vi "Timeout AutoKAL.vi"(6 "Aktionen":T1) -> (0 "Timeout":bool, 2 "Verstrichene Zeit":dbl)   [LabVIEW 2020, in "Auto Kalibrieren.lvlib"]
uses:
  Auto Kalibrieren.lvlib
  Aktionen Timeout.ctl
  Aktionen FGV Zustand Kalibrierung.ctl
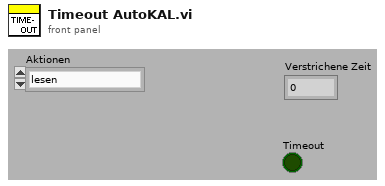
[diagram p1: front panel]
types:
  T1 = typedef "Auto Kalibrieren.lvlib/Aktionen Timeout.ctl" = enum16{"lesen", "init", "prüfen"}
  T2 = typedef "Auto Kalibrieren.lvlib/Aktionen FGV Zustand Kalibrierung.ctl" = enum16{"lesen", "LÖSCHEN", "Hintergrund fertig", "Nullpunkt NDIR CO lo", "Endpunkt NDIR CO lo", "Nullpunkt NDIR CO hi", "Endpunkt NDIR CO hi", "Nullpunkt NDIR CO2 lo", "Endpunkt NDIR CO2 lo", "Nullpunkt FID CH4", "Endpunkt FID CH4", "Nullpunkt FID THC", "Endpunkt FID THC", "Nullpunkt PMA", "Endpunkt PMA", "Fehler FT-IR", "Fehler NDIR lo", "Fehler FID CH4", "Fehler FID THC", "Fehler PMA", "TIMEOUT"}
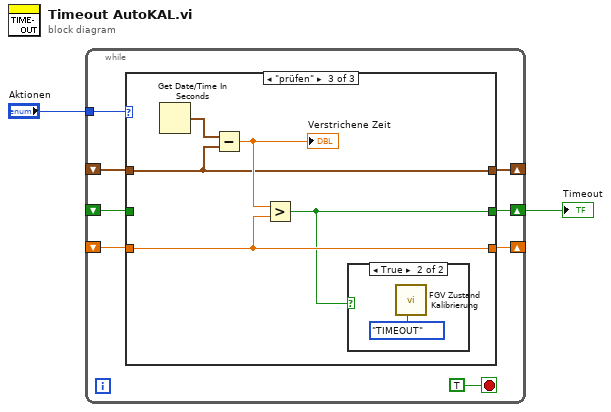
[diagram p0: block diagram]
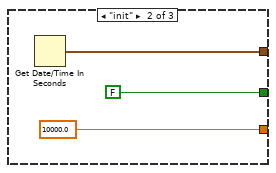
[diagram p3: hidden frame]
diagram:
  n1 = while {
    tunnel: "Aktionen" -> [w9]
    shift-right: [w8] -> _
    shift-left: _ -> [w7]
    shift-right: [w5] -> _
    shift-left: _ -> [w6]
    shift-right: [w4] -> w1
    shift-left: _ -> [w3]
    stop <- TRUE stop-if-true
    n2 = case shown="\"prüfen\"" w9 {
      tunnel: [w13 w16 w18] -> w8
      tunnel: w7 -> [w13 _ w18]
      tunnel: w6 -> [w12 _ w19]
      tunnel: [w12 sgl 10000.0 w19] -> w5
      tunnel: [w11 FALSE w17] -> w4
      tunnel: w3 -> [w11 _ _]
      frame "lesen", Default {
      }
      frame "init" {
        n3 = Get Date/Time In Seconds() -> (seconds since 1Jan1904=w16:timestamp)
      }
      frame "prüfen" {
        n4 = Get Date/Time In Seconds() -> (seconds since 1Jan1904=w21:timestamp)
        n5 = Subtract(x=w21, y=w18) -> (x-y=w20:dbl)
        "Verstrichene Zeit" <- w20
        n6 = Greater?(x=w20, y=w19) -> (0:w17:bool)
        n7 = case shown="True" w17 {
          frame False {
          }
          frame True {
            n8 = call "FGV Zustand Kalibrierung.vi"("Aktionen"=Aktionen_FGV_Zustand_Kalibrierung."TIMEOUT" ("Enum")) -> ()  [unwired: 9 in, 2 out]
          }
        }
      }
    }
  }
  "Timeout" <- w1
